vi "Initialization VI.vi"(8 "error in (no error)":errorcluster, 10 "Custom XML":string, 11 "Device Item Ref in":T1 format="%.0x") -> (0 "error out":errorcluster, 3 "Device Item Ref out":T1 format="%.0x")   [LabVIEW 2021, in "Large Number Operation System Explorer.lvlib"]
uses:
  Large Number Operation System Explorer.lvlib
  <vilib>/NI VeriStand/Custom Device API/Custom Device Item Ref.ctl
  <vilib>/NI VeriStand/Custom Device API/Custom Device Channel.ctl
  <vilib>/NI VeriStand/Custom Device API/Custom Device Channel Type.ctl
  <vilib>/NI VeriStand/Custom Device API/Set Item Property (U16).vi
  <vilib>/NI VeriStand/Custom Device API/Set Item Property (String).vi
  <vilib>/NI VeriStand/Custom Device API/Custom Device API.lvlib
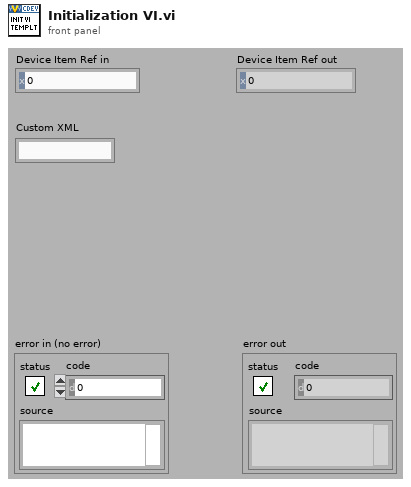
[diagram p1: front panel]
types:
  T1 = typedef "Custom Device API.lvlib/Custom Device Item Ref.ctl" = u64
  T2 = typedef "Custom Device API.lvlib/Custom Device Channel.ctl" = cluster{"Type":T3, "Units":string, "Default Value":dbl, "Faultable":bool, "Scalable":bool}
  T3 = typedef "Custom Device API.lvlib/Custom Device Channel Type.ctl" = enum16{"Input", "Output"}
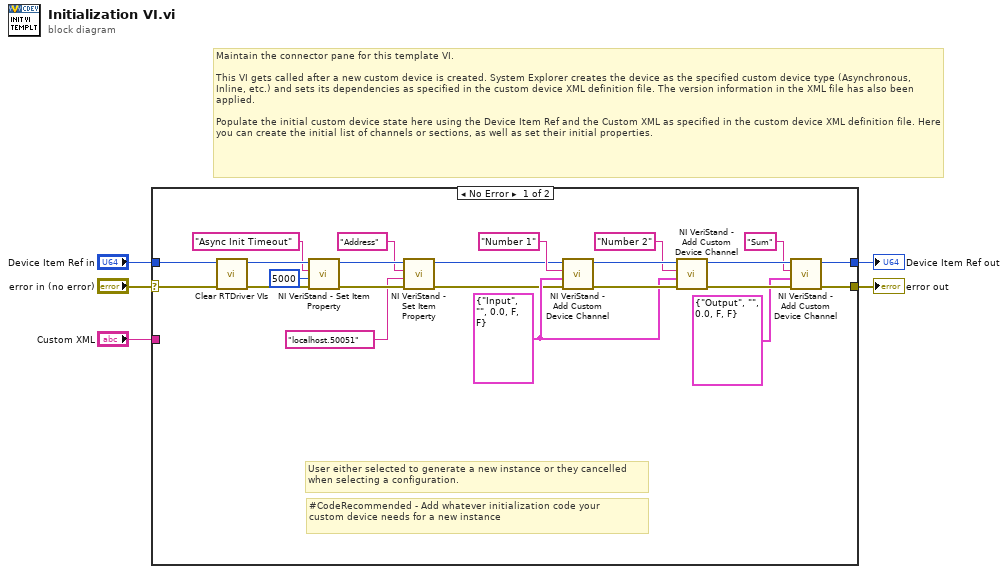
[diagram p0: block diagram]
diagram:
  # "Maintain the connector pane for this template VI.\n\nThis VI gets called after a new custom device is created. System Explorer creates the device as the specified custom device type (Asynchronous, Inline, etc.) and sets its dependencies as specified in the custom device XML definition file. The version information in the XML file has also been applied.\n\nPopulate the initial custom device state here using the Device Item Ref and the Custom XML as specified in the custom device XML definition file. Here you can create the initial list of channels or sections, as well as set their initial properties."
  n1 = case shown="No Error" "error in (no error)" {
    selector: "error in (no error)" -> [w27 w30]
    tunnel: [w15 w30] -> w5
    tunnel: [w16 w29] -> w3
    tunnel: "Device Item Ref in" -> [w28 w29]
    tunnel: "Custom XML" -> [_ _]
    frame No Error {
      w13 = T2 {"Type"=enum."Input", "Units"="", "Default Value"=0.0, "Faultable"=FALSE, "Scalable"=FALSE} ("Channel")
      # "#CodeRecommended - Add whatever initialization code your\ncustom device needs for a new instance"
      # "User either selected to generate a new instance or they cancelled\nwhen selecting a configuration."
      n2 = call "Clear RTDriver VIs.vi"("error in (no error)"=w27, "Device Item Ref in in"=w28) -> ("error out"=w25:errorcluster, "Device Item Ref out"=w26:T1)  [unwired: 8 in]
      n3 = call-poly <vilib>:"NI VeriStand - Set Item Property.vi"("error in (no error)"=w25, "Value"=u16 5000, "Property Name"="Async Init Timeout", "Item Ref in"=w26) -> ("error out"=w9:errorcluster, "Item Ref out"=w11:T1)  [unwired: 5 in, 1 out]
      n4 = call-poly <vilib>:"NI VeriStand - Set Item Property.vi"("error in (no error)"=w9, "Value"="localhost.50051", "Property Name"="Address", "Item Ref in"=w11) -> ("error out"=w6:errorcluster, "Item Ref out"=w7:T1)  [unwired: 5 in, 1 out]
      n5 = call <vilib>:"NI VeriStand - Add Custom Device Channel.vi"("error in (no error)"=w6, "Channel"=w13, "Channel Name"="Number 1", "Parent Ref in"=w7) -> ("error out"=w21:errorcluster, "Parent Ref out"=w22:T1)  [unwired: 4 in, 2 out]
      n6 = call <vilib>:"NI VeriStand - Add Custom Device Channel.vi"("error in (no error)"=w21, "Channel"=w13, "Channel Name"="Number 2", "Parent Ref in"=w22) -> ("error out"=w17:errorcluster, "Parent Ref out"=w18:T1)  [unwired: 4 in, 2 out]
      n7 = call <vilib>:"NI VeriStand - Add Custom Device Channel.vi"("error in (no error)"=w17, "Channel"=T2 {"Type"=enum."Output", "Units"="", "Default Value"=0.0, "Faultable"=FALSE, "Scalable"=FALSE}, "Channel Name"="Sum", "Parent Ref in"=w18) -> ("error out"=w15:errorcluster, "Parent Ref out"=w16:T1)  [unwired: 4 in, 2 out]
    }
    frame Error {
    }
  }
  "error out" <- w5
  "Device Item Ref out" <- w3
